vi "NicmosSwichToTriggeredMode.vi"(6 "error in (no error)":errorcluster caption="entrée d'erreur") -> (0 "error out":errorcluster caption="sortie d'erreur")   [LabVIEW 2009]
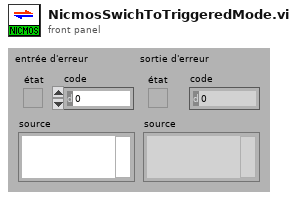
[diagram p1: front panel]
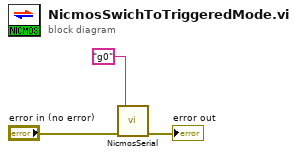
[diagram p0: block diagram]
diagram:
  n1 = call "NicmosSerial.vi"("error in"="error in (no error)", "Command"="g0") -> ("error out"=→"error out":errorcluster)  [unwired: 3 in, 1 out]
